vi "BLM Init.vi"(3 "error in (no error)":errorcluster, 4 "Baud Rate":u32=9600, 5 "Motor Address":string="0", 6 "Port Address":refnum<visa-resource-name>) -> (0 "error out":errorcluster, 1 "Response":string, 2 "Port Address Out":refnum<visa-resource-name>)   [LabVIEW 2019]
uses:
  Serial Instruments/Serial Support VISA.llb/Serial Actions.ctl
  BLM_IgnoreAlarms.vi
panel:
  in  "Limit Switches":bool
  in  "Velocity":dbl=0.42 min=0.0042 max=0.42 step=0.0042
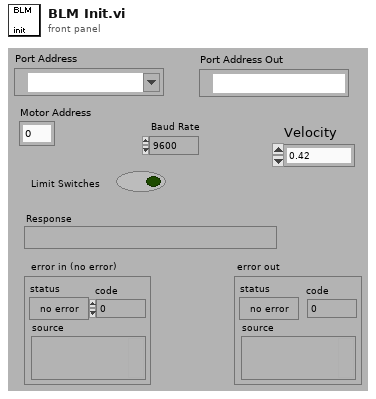
[diagram p1: front panel]
types:
  T1 = cluster{"flow control":enum16{"None", "XON/XOFF", "RTS/CTS"}, "baud rate":u32, "data bits":u16, "Stop Bits":u16, "parity (0:none)":enum16{"None", "Odd", "Even", "Mark", "Space"}, "Transmit Buffer Size":u32, "Receive Buffer Size":u32}
  T2 = typedef "Serial Actions.ctl" = enum16{"Init", "Break", "Clear Buffer", "Write", "Read", "N Bytes", "Lock", "Unlock", "Close"}
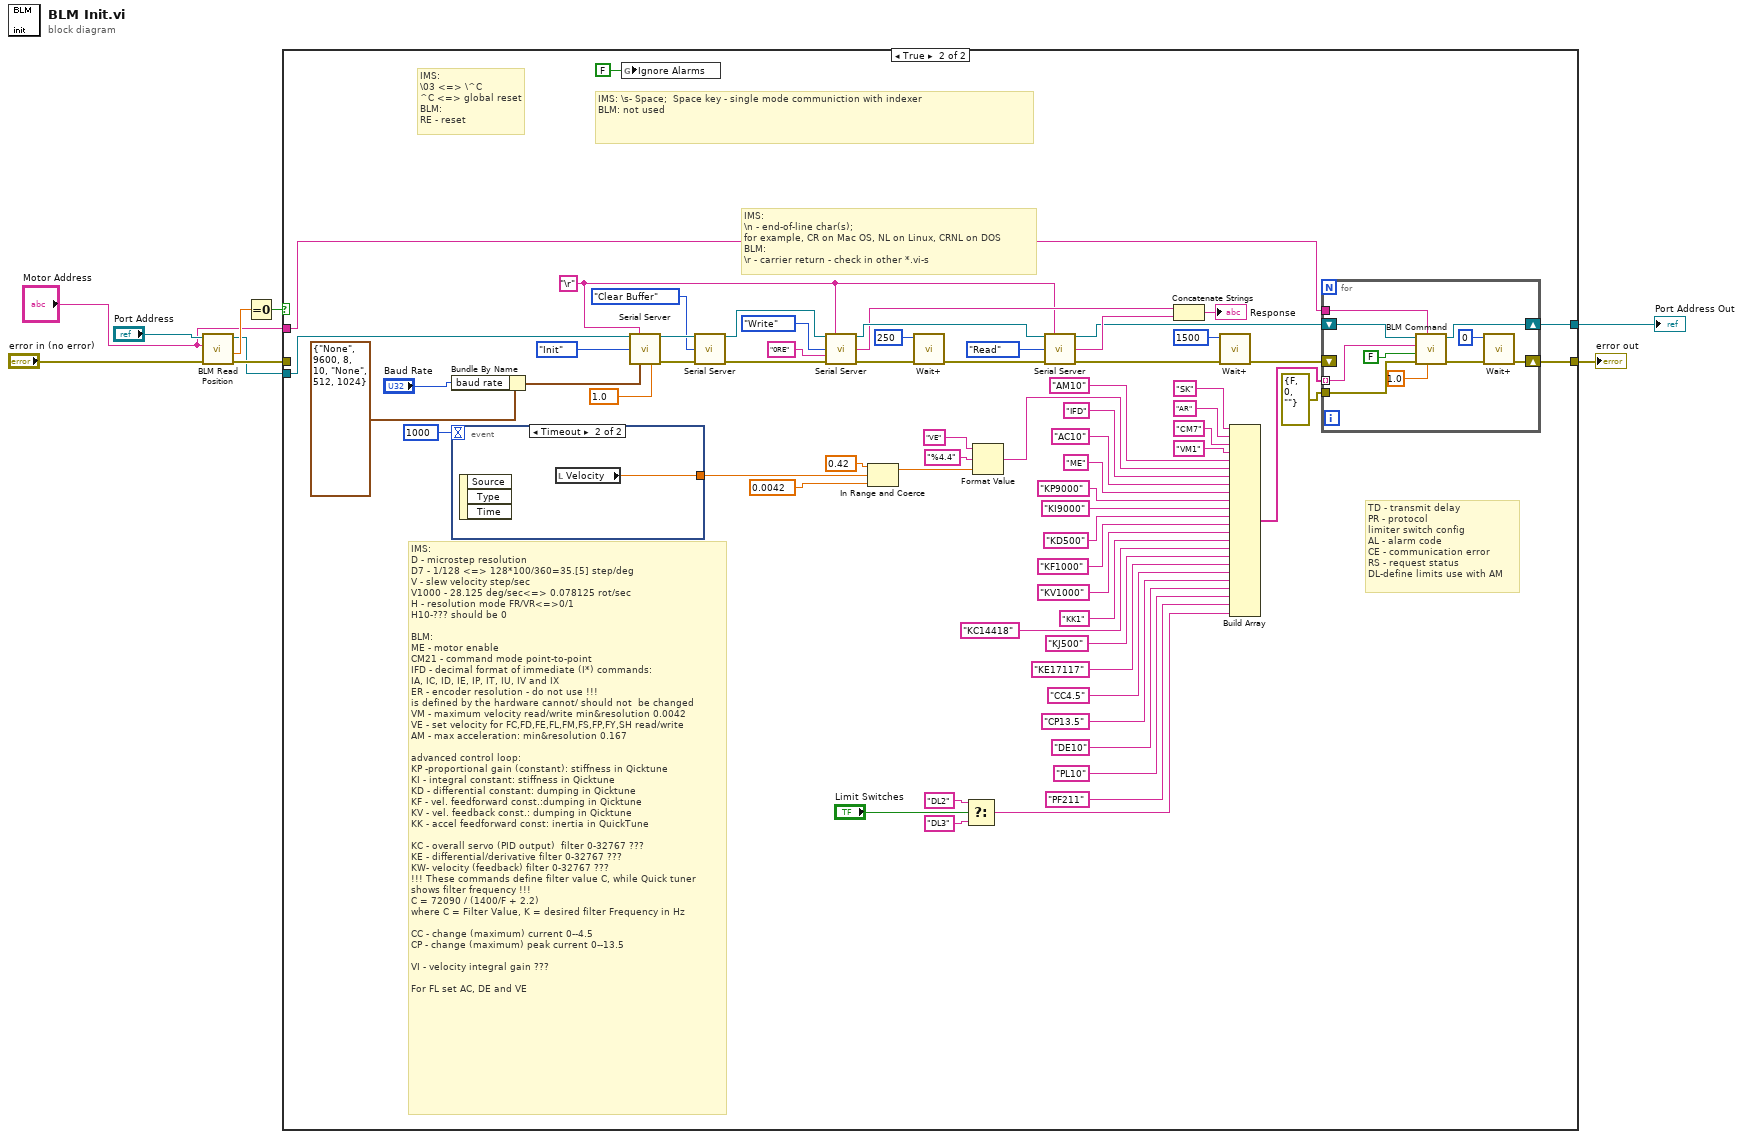
[diagram p0: block diagram]
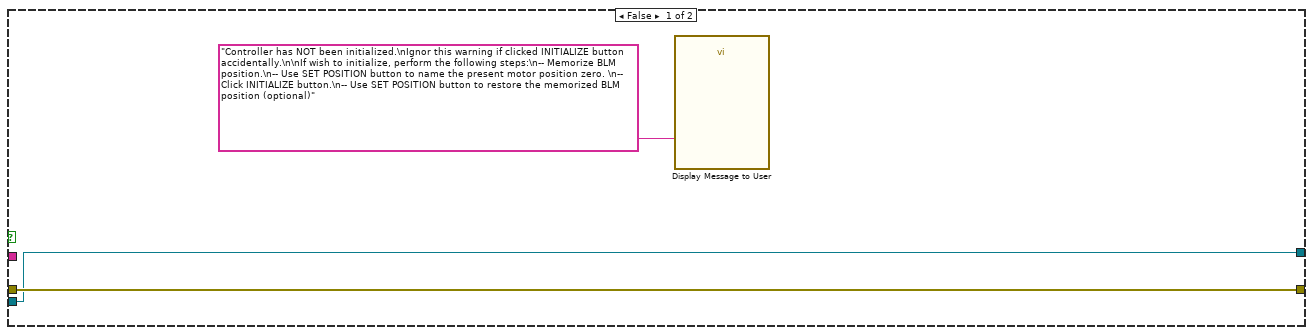
[diagram p2: hidden frame]
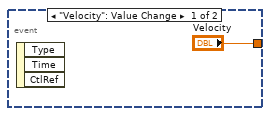
[diagram p3: hidden frame]
diagram:
  n1 = call "BLM Read Position.vi"("error in (no error)"="error in (no error)", "Motor Address"="Motor Address", "Port Address"="Port Address") -> ("error out"=w8:errorcluster, "Response"=w9:dbl, "Port Address Out"=w1:refnum<visa-resource-name>)  [unwired: 1 in, 1 out]
  n2 = Equal To 0?(x=w9) -> (x = 0?=w4:bool)
  n3 = case shown="True" w4 {
    tunnel: w8 -> [w12 _]
    tunnel: w1 -> [w10 w78]
    tunnel: [w12 w77] -> w5
    tunnel: "Motor Address" -> [_ w18]
    tunnel: [w10 w17] -> w2
    frame False {
      n4 = call "Display Message to User"("Message"="Controller has NOT been initialized.\nIgnor this warning if clicked INITIALIZE button accidentally.\n\nIf wish to initialize, perform the following steps:\n-- Memorize BLM position.\n-- Use SET POSITION button to name the present motor position zero. \n-- Click INITIALIZE button.\n-- Use SET POSITION button to restore the memorized BLM position (optional)" ("message")) -> ()  [unwired: 9 in, 2 out]
    }
    frame True {
      w53 = "\r" ("EOT Chars (cr/lf)")
      # "IMS:\nD - microstep resolution\nD7 - 1/128 <=> 128*100/360=35.[5] step/deg\nV - slew velocity step/sec\nV1000 - 28.125 deg/sec<=> 0.078125 rot/sec\nH - resolution mode FR/VR<=>0/1\nH10-??? should be 0\n\nBLM:\nME - motor enable\nCM21 - command mode point-to-point\nIFD - decimal format of immediate (I*) commands:\nIA, IC, ID, IE, IP, IT, IU, IV and IX\nER - encoder resolution - do not use !!!\nis defined by the hardware cannot/ should not  be changed\nVM - maximum velocity read/write min&resolution 0.0042\nVE - set velocity for FC,FD,FE,FL,FM,FS,FP,FY,SH read/write\nAM - max acceleration: min&resolution 0.167\n\nadvanced control loop:\nKP -proportional gain (constant): stiffness in Qicktune\nKI - integral constant: stiffness in Qicktune\nKD - differential constant: dumping in Qicktune \nKF - vel. feedforward const.:dumping in Qicktune \nKV - vel. feedback const.: dumping in Qicktune \nKK - accel feedforward const: inertia in QuickTune\n\nKC - overall servo (PID output)  filter 0-32767 ???\nKE - differential/derivative filter 0-32767 ???\nKW- velocity (feedback) filter 0-32767 ???\n!!! These commands define filter value C, while Quick tuner \nshows filter frequency !!!\nC = 72090 / (1400/F + 2.2)\nwhere C = Filter Value, K = desired filter Frequency in Hz\n\nCC - change (maximum) current 0--4.5\nCP - change (maximum) peak current 0--13.5\n\nVI - velocity integral gain ???\n\nFor FL set AC, DE and VE"
      # "IMS: \\s- Space;  Space key - single mode communiction with indexer\nBLM: not used"
      # "IMS:\n\\n - end-of-line char(s); \nfor example, CR on Mac OS, NL on Linux, CRNL on DOS\nBLM:\n\\r - carrier return - check in other *.vi-s"
      # "TD - transmit delay\nPR - protocol\nlimiter switch config\nAL - alarm code\nCE - communication error\nRS - request status\nDL-define limits use with AM"
      # "IMS:\n\\03 <=> \\^C \n^C <=> global reset\nBLM:\nRE - reset"
      n5 = Bundle By Name(cluster=T1 {"flow control"=enum."None", "baud rate"=9600, "data bits"=8, "Stop Bits"=10, "parity (0:none)"=enum."None", "Transmit Buffer Size"=512, "Receive Buffer Size"=1024} ("Port Parameters"), "baud rate"="Baud Rate") -> (w66:T1)
      n6 = event shown="[1] Timeout" {
        selector: _ -> [_ _]
        dyn-events: _ -> [_ _]
        timeout: 1000 -> [_ _]
        tunnel: ["Velocity" w80] -> w38
        event "Velocity": Value Change {
          n7 = event-data() -> ()  [unwired: 1 in, 3 out]
        }
        event Timeout {
          n8 = event-data() -> ()  [unwired: 1 in, 3 out]
          n9 = local read "Velocity"() -> (w80:dbl)
        }
      }
      n10 = global write "BLM_IgnoreAlarms.vi" "Ignore Alarms"(FALSE ("Ignore Alarms")) -> ()
      n11 = call "Serial Server.vi"("VISA Resource Name"=w78, "EOT Chars (cr/lf)"=w53, "Action"=Serial_Actions."Init", "Port Parameters"=w66, "Timeout Limit(sec)"=1.0 ("Timeout Limit")) -> ("dup VISA Resource Name"=w65:refnum<visa-resource-name>, "error out"=w62:errorcluster)  [unwired: 6 in, 3 out]
      n12 = call "Serial Server.vi"("VISA Resource Name"=w65, "Action"=Serial_Actions."Clear Buffer", "error in (no error)"=w62) -> ("dup VISA Resource Name"=w76:refnum<visa-resource-name>, "error out"=w75:errorcluster)  [unwired: 8 in, 3 out]
      n13 = call "Serial Server.vi"("VISA Resource Name"=w76, "EOT Chars (cr/lf)"=w53, "Action"=Serial_Actions."Write", "String To Send"="0RE" ("Command"), "error in (no error)"=w75) -> ("dup VISA Resource Name"=w56:refnum<visa-resource-name>, "Serial Read"=w55:string, "error out"=w73:errorcluster)  [unwired: 6 in, 2 out]
      n14 = In Range and Coerce(upper limit=0.42 ("x"), x=w38, lower limit=0.0042) -> (coerced(x)=w35:dbl)  [unwired: 1 out]
      n15 = call "Wait+.vi"("Error In"=w73, "milliseconds to wait"=u32 250) -> ("Error Out"=w54:errorcluster)  [unwired: 4 in, 1 out]
      n16 = Select(t="DL2" ("element"), s="Limit Switches", f="DL3" ("element")) -> (s? t:f=w15:string)
      n17 = Format Value(string ("")="VE", format string="%4.4", value (0)=w35) -> (output string=w34:string)
      n18 = call "Serial Server.vi"("VISA Resource Name"=w56, "EOT Chars (cr/lf)"=w53, "Action"=Serial_Actions."Read", "error in (no error)"=w54) -> ("dup VISA Resource Name"=w26:refnum<visa-resource-name>, "Serial Read"=w71:string, "error out"=w21:errorcluster)  [unwired: 7 in, 2 out]
      n19 = Concatenate Strings(w55, w71) -> (→"Response":string)
      n20 = call "Wait+.vi"("Error In"=w21, "milliseconds to wait"=u32 1500) -> ("Error Out"=w20:errorcluster)  [unwired: 4 in, 1 out]
      n21 = Build Array("SK" ("element"), "AR" ("element"), "CM7", "VM1", "AM10" ("element"), w34, "IFD" ("element"), "AC10" ("element"), "ME" ("element"), "KP9000" ("element"), "KI9000" ("element"), "KD500" ("element"), "KF1000" ("element"), "KV1000" ("element"), "KK1" ("element"), "KC14418" ("element"), "KJ500" ("element"), "KE17117" ("element"), "CC4.5" ("element"), "CP13.5" ("element"), "DE10" ("element"), "PL10" ("element"), "PF211" ("element"), w15) -> (w59:string[])
      n22 = for {
        shift-right: [w82] -> w77
        shift-left: w20 -> [_]
        tunnel: w59 -> [w89] mode=indexing
        tunnel: errorcluster {"status"=FALSE, "code"=0, "source"=""} ("error in (no error)") -> [w85]
        tunnel: w18 -> [w83]
        shift-right: [w81] -> w17
        shift-left: w26 -> [w88]
        n23 = call "BLM Command.vi"("Timeout Limit"=sgl 1.0, "Motor Address"=w83, "error in (no error)"=w85, "Read Echo?"=FALSE, "Command"=w89, "Port Address"=w88) -> ("error out"=w87:errorcluster, "Port Address Out"=w81:refnum<visa-resource-name>)  [unwired: 3 out]
        n24 = call "Wait+.vi"("Error In"=w87, "milliseconds to wait"=u32 0) -> ("Error Out"=w82:errorcluster)  [unwired: 4 in, 1 out]
      }
    }
  }
  "error out" <- w5
  "Port Address Out" <- w2
